vi "Read Channel Data.vi"(8 "error in (no error)":errorcluster, 11 "Software Lock-in in":refnum<class "Software Lock-in.lvclass">) -> (0 "error out":errorcluster, 1 "Finished":bool, 2 "Data":dbl[](array[numeric]), 3 "Software Lock-in out":refnum<class "Software Lock-in.lvclass">)   [LabVIEW 2020, in "Software Lock-in.lvclass"]
uses:
  Software Lock-in.lvclass
  Software Lock-in.lvclass/Software Lock-in.ctl
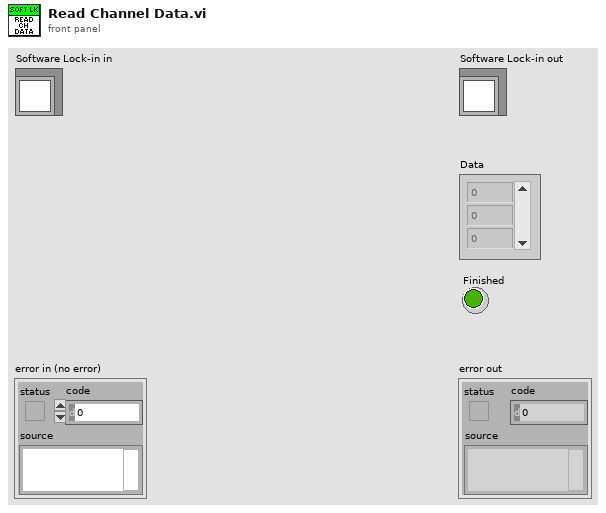
[diagram p1: front panel]
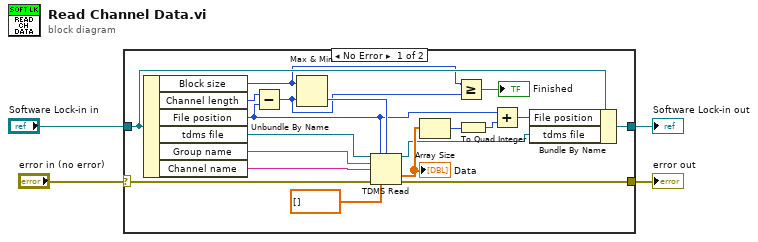
[diagram p0: block diagram]
diagram:
  n1 = case shown="No Error" "error in (no error)" {
    selector: "error in (no error)" -> [w19 w25]
    tunnel: [w15 w25] -> w3
    tunnel: [w14 w24] -> w1
    tunnel: "Software Lock-in in" -> [w23 w24]
    frame No Error {
      n2 = Unbundle By Name(w23) -> ("Block size"=w7:i64, "Channel length"=w21:i64, "File position"=w11:i64, "tdms file"=w22:refnum<k34>, "Group name"=w18:string, "Channel name"=w17:string)
      n3 = Subtract(x=w21, y=w11) -> (x-y=w6:i64)
      n4 = Max & Min(x=w7, y=w6) -> (min(x,y)=w20:i64)  [unwired: 1 out]
      n5 = TDMS Read(0:w22, 1:w11, 2:w20, 5:w18, 7:w17, 11:w19, 12:dbl[] []) -> (4:w9:refnum<k34>, 10:w13:dbl[], 15:w15:errorcluster)  [unwired: 1 in, 3 out]
      "Data" <- w13
      n6 = Array Size(array=w13) -> (size(s)=w12:i32)
      n7 = Greater Or Equal?(x=w7, y=w6) -> (x >= y?=→"Finished":bool)
      n8 = To Quad Integer(1:w12) -> (0:w8:i64)
      n9 = Add(x=w11, y=w8) -> (x+y=w10:i64)
      n10 = Bundle By Name(cluster=w23, "File position"=w10, "tdms file"=w9) -> (w14:refnum<class "Software Lock-in.lvclass">)
    }
    frame Error {
    }
  }
  "error out" <- w3
  "Software Lock-in out" <- w1
